vi "Write inPositionAzIsTrue.vi"(8 "error in (no error)":errorcluster, 10 "inPositionAzIsTrue":bool, 11 "TCSTcsStatus in":refnum<class "TCSTcsStatus.lvclass">) -> (0 "error out":errorcluster, 3 "TCSTcsStatus out":refnum<class "TCSTcsStatus.lvclass">)   [LabVIEW 2014, in "TCSDataDefinitions.lvlib" / "TCSPublicStatus.lvlib" / "TCSTcsStatus.lvclass"]
uses:
  TCSTcsStatus.lvclass
  TCSTcsStatus.lvclass/TCSTcsStatus.ctl
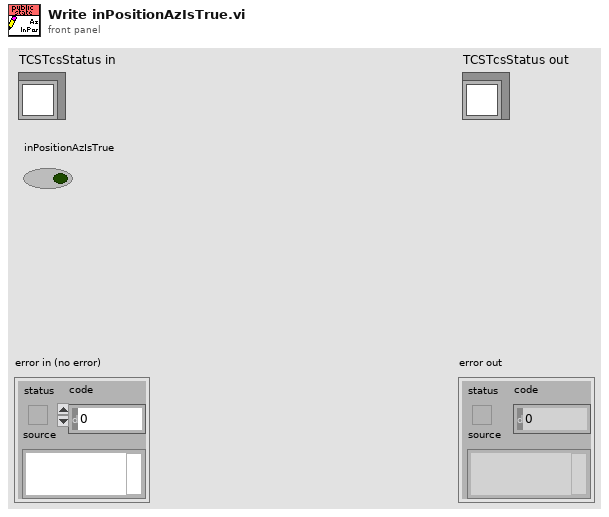
[diagram p1: front panel]
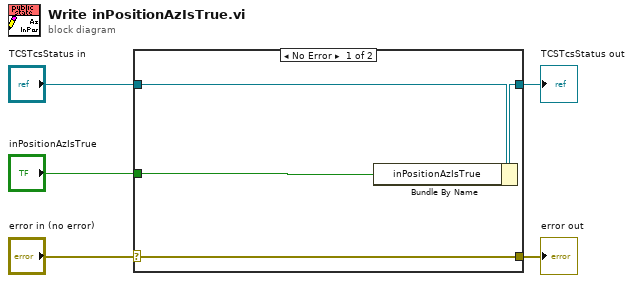
[diagram p0: block diagram]
diagram:
  n1 = case shown="No Error" "error in (no error)" {
    selector: "error in (no error)" -> [w9 w10]
    tunnel: [w9 w10] -> w4
    tunnel: [w7 w11] -> w2
    tunnel: "TCSTcsStatus in" -> [w8 w11]
    tunnel: "inPositionAzIsTrue" -> [w6 _]
    frame No Error {
      n2 = Bundle By Name(cluster=w8, "inPositionAzIsTrue"=w6) -> (w7:refnum<class "TCSTcsStatus.lvclass">)
    }
    frame Error {
    }
  }
  "error out" <- w4
  "TCSTcsStatus out" <- w2
